vi "S7_Read_Write_Data_TCP.vi"(0 "TCP Connection Ref":refnum<k5>, 1 "Read / Write":u8(ring)=4 items=["Read"=4, "Write"=5], 5 "Address Areas":u8(ring)=128 format="%02x" items=["I/O (P)"=128, "Input (I)"=129, "Output (Q)"=130, "Bit Memory (M)"=131, "Data (DB)"=132, "Instance Data (DI)"=133, "Local Data (L)"=134, "Predecessor Local Data (VL)"=135], 7 "Start Address (bytes)":u32=131, 9 "Data Block #":u16=1, 11 "error in":errorcluster, 12 "Write Data":i32 format="%08x", 13 "Length (bytes)":u16=1, 14 "Timeout":u32=1000) -> (4 "TCP Connection Ref Out":refnum<k5>, 6 "Data Valid":bool, 10 "Data Read":u8[](array[numeric]), 15 "error out":errorcluster)   [LabVIEW 2017, in "S7 TCP.lvlib"]
uses:
  S7 TCP.lvlib
panel:
  # "Max Length = 222\n(corresponds to total\nPDU length of 240; 18\nvalues in PDU & data\nheader)"
  # "Data Block only valid\nwhen reading / writing \n\"Data (DB)\" Address Area"
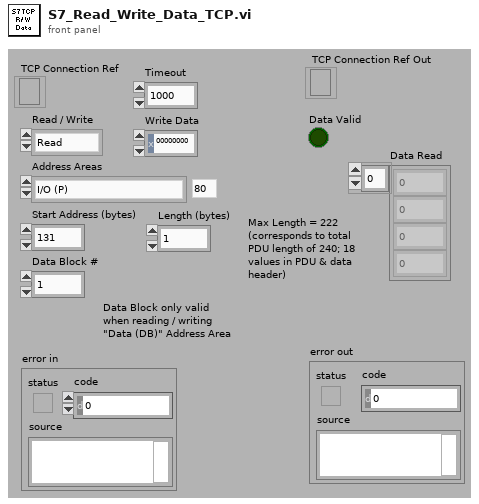
[diagram p1: front panel]
types:
  T1 = enum16{"Standard", "Buffered", "CRLF", "Immediate"}
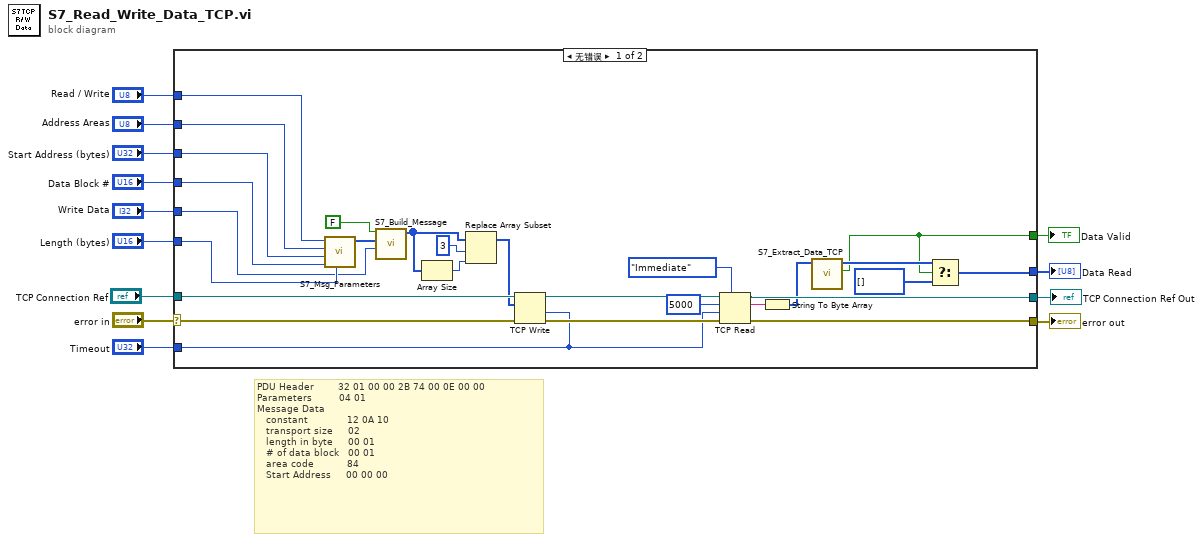
[diagram p0: block diagram]
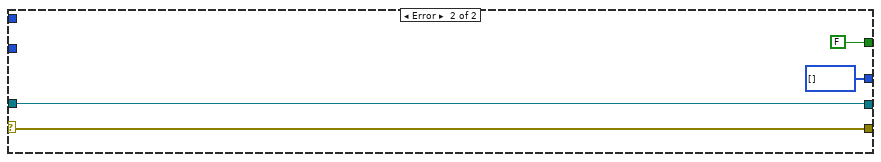
[diagram p2: hidden frame]
diagram:
  # "PDU Header        32 01 00 00 2B 74 00 0E 00 00 \nParameters         04 01 \nMessage Data       \n   constant             12 0A 10\n   transport size     02\n   length in byte     00 01\n   # of data block   00 01\n   area code           84\n   Start Address     00 00 00"
  n1 = case shown="无错误" "error in" {
    selector: "error in" -> [w30 w43]
    tunnel: "TCP Connection Ref" -> [w31 w44]
    tunnel: "Timeout" -> [w24 _]
    tunnel: "Length (bytes)" -> [w39 _]
    tunnel: "Write Data" -> [w14 _]
    tunnel: "Data Block #" -> [w38 _]
    tunnel: "Start Address (bytes)" -> [w37 _]
    tunnel: "Address Areas" -> [w36 _]
    tunnel: "Read / Write" -> [w19 _]
    tunnel: [w27 w44] -> w1
    tunnel: [w26 w43] -> w6
    tunnel: [w20 u8[] [] ("f")] -> w5
    tunnel: [w32 FALSE ("Data Valid")] -> w4
    frame No Error {
      n2 = call "S7_Msg_Parameters.vi"("Length (bytes)"=w39, "Data Block #"=w38, "Start Address (bytes)"=w37, "Address Areas"=w36, "Read / Write"=w19) -> ("Message Parameters"=w40:u8[])  [unwired: 6 out]
      n3 = call "S7_Build_Message.vi"("Write Data"=w14, "Parameters"=w40, "Exchange PDU"=FALSE) -> ("S7 Ethernet Data"=w15:u8[])  [unwired: 8 out]
      n4 = Array Size(array=w15) -> (size(s)=w16:i32)
      n5 = Replace Array Subset(array=w15, new element=w16, index=3) -> (w18:u8[])
      n6 = TCP Write(connection ID=w31, data in=w18, error in (no error)=w30, 9:w24) -> (connection ID out=w29:refnum<k5>, error out=w28:errorcluster)  [unwired: 1 out]
      n7 = TCP Read(connection ID=w29, bytes to read=5000, error in (no error)=w28, 7:T1."Immediate" ("mode (standard)"), 9:w24) -> (connection ID out=w27:refnum<k5>, data out=w25:string, error out=w26:errorcluster)
      n8 = String To Byte Array(string=w25) -> (unsigned byte array=w21:u8[])
      n9 = call "S7_Extract_Data_TCP.vi"("Data Recieved"=w21) -> ("Data Valid"=w32:bool, "Data"=w34:u8[])  [unwired: 9 out]
      n10 = Select(t=w34, s=w32, f=u8[] []) -> (s? t:f=w20:u8[])
    }
    frame Error {
    }
  }
  "error out" <- w6
  "Data Read" <- w5
  "Data Valid" <- w4
  "TCP Connection Ref Out" <- w1
